vi "xijk_make_laser.vi"(9 "Broadness of laser (nm)":u16, 11 "Wavelength of laser (nm)":u16) -> (1 "laser_y":dbl[](array[numeric]), 3 "laser_x":i16[](array[numeric]))   [LabVIEW 2010]
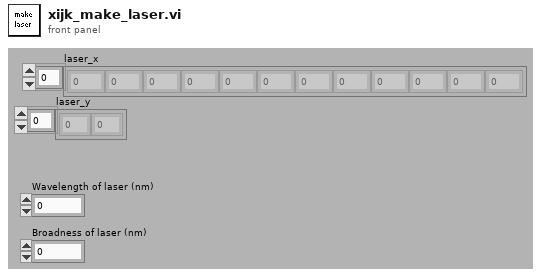
[diagram p1: front panel]
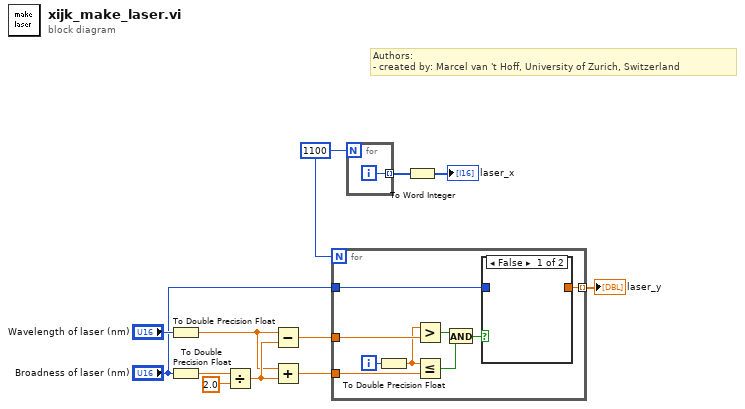
[diagram p0: block diagram]
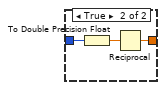
[diagram p2: hidden frame]
diagram:
  w1 = 1100 ("taille de la dimension")
  # "Authors: \n- created by: Marcel van 't Hoff, University of Zurich, Switzerland"
  n1 = To Double Precision Float(number="Wavelength of laser (nm)") -> (double precision float=w5:dbl)
  n2 = To Double Precision Float(number="Broadness of laser (nm)") -> (double precision float=w6:dbl)
  n3 = Divide(x=w6, y=2.0) -> (x/y=w10:dbl)
  n4 = Subtract(x=w5, y=w10) -> (x-y=w8:dbl)
  n5 = Add(x=w5, y=w10) -> (x+y=w7:dbl)
  n6 = for {
    N: w1 -> [_]
    tunnel: [w16] -> w9 mode=indexing
    tunnel: w8 -> [w18]
    tunnel: w7 -> [w17]
    tunnel: "Broadness of laser (nm)" -> [w14]
    i -> [w15]
    n7 = To Double Precision Float(number=w15) -> (double precision float=w13:dbl)
    n8 = Greater?(x=w13, y=w18) -> (0:w21:bool)
    n9 = Less Or Equal?(x=w13, y=w17) -> (x <= y?=w20:bool)
    n10 = And(x=w21, y=w20) -> (x .and. y?=w19:bool)
    n11 = case shown="False" w19 {
      tunnel: [_ w24] -> w16
      tunnel: w14 -> [_ w22]
      frame False {
      }
      frame True {
        n12 = To Double Precision Float(number=w22) -> (double precision float=w23:dbl)
        n13 = Reciprocal(x=w23) -> (1/x=w24:dbl)
      }
    }
  }
  "laser_y" <- w9
  n14 = for {
    N: w1 -> [_]
    tunnel: [w25] -> w3 mode=indexing
    i -> [w25]
  }
  n15 = To Word Integer(number=w3) -> (16bit integer=→"laser_x":i16[])
